vi "SUB_Calibration_by_KH_170117.vi"(11 "Test Data table":string[][](table)=[["-", "-", "5", "10", "20.025", "29.975", "39.9"], ["-", "-", "-", "-", "-", "-", "-"], ["-", "-", "-", "-", "-", "-", "-"], ["-", "-", "-", "-", "-", "-", "-"], ["-", "-", "109.9", "248.8", "515.2", "773.0", "1024.30"], ["-", "-", "-", "-", "-", "-", "-"], ["-", "-", "-", "-", "-", "-", "-"], ["-", "-", "-", "-", "-", "-", "-"], ["-", "-", "59.10", "162.20", "378.80", "615.60", "863.10"]]) -> (2 "Calibration Parameter-R":T1 {"lb offset" format="%#_13g"; "y intercept" format="%#_13g"; "Scale" format="%#_13g"; "Linear fit" format="%#_13g"}, 3 "Calibration Parameter-L":T1 {"lb offset" format="%#_13g"; "y intercept" format="%#_13g"; "Scale" format="%#_13g"; "Linear fit" format="%#_13g"})   [LabVIEW 2015]
uses:
  <vilib>/Analysis/6fits.llb/Curve Fitting Criteria.ctl
  <vilib>/Analysis/NI_AALPro.lvlib
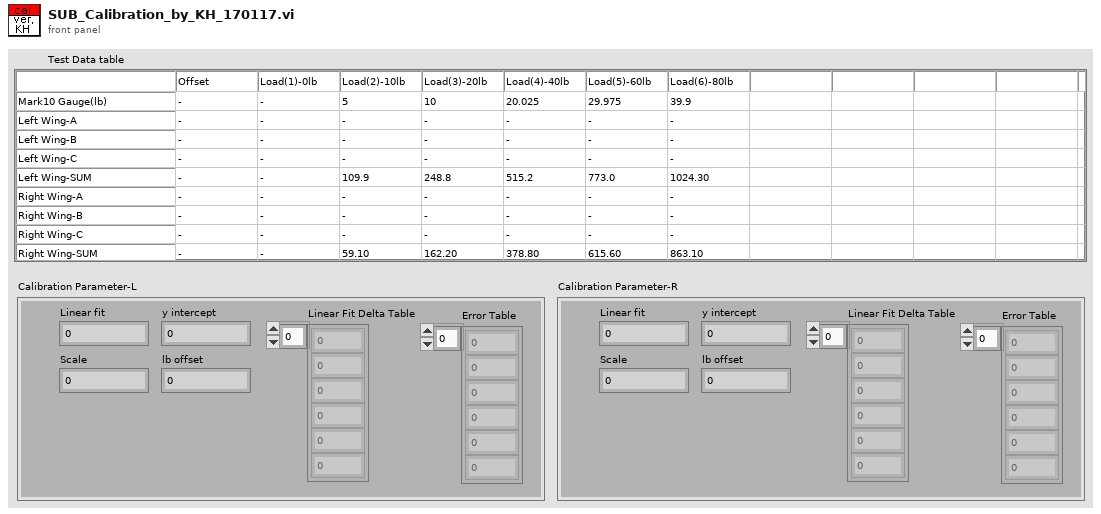
[diagram p1: front panel]
types:
  T1 = cluster{"Linear fit":dbl, "Scale":dbl, "Error Table":dbl[], "y intercept":dbl, "lb offset":dbl, "Linear Fit Delta Table":dbl[]}
  T2 = typedef "NI_AALPro.lvlib/Curve Fitting Criteria.ctl" = u16
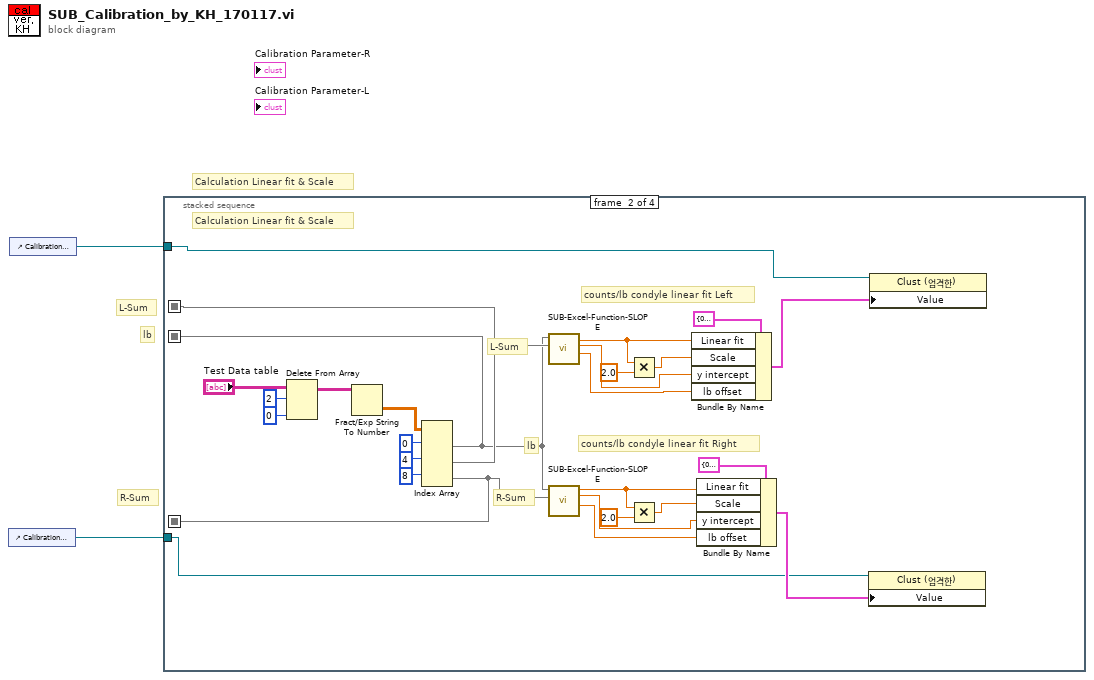
[diagram p0: block diagram]
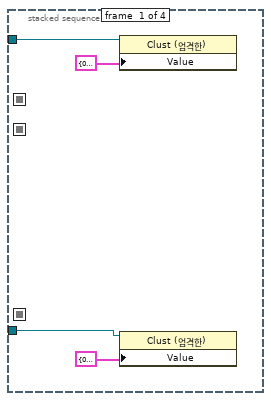
[diagram p2: hidden frame]
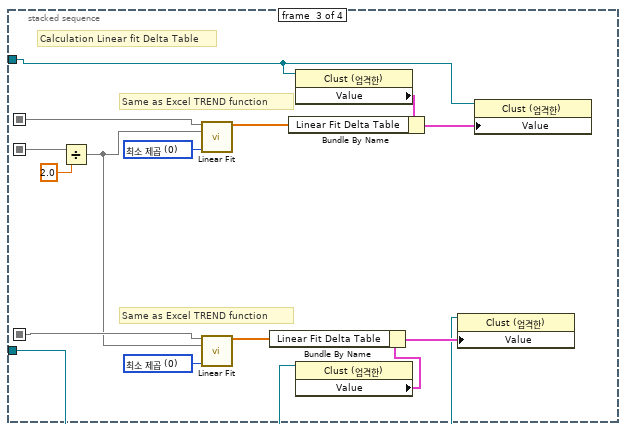
[diagram p3: hidden frame]
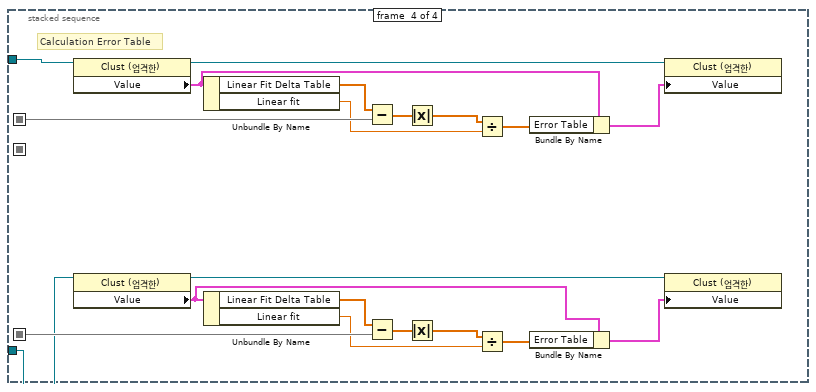
[diagram p4: hidden frame]
diagram:
  # "Calculation Linear fit & Scale"
  # "lb"
  # "R-Sum"
  # "L-Sum"
  n1 = control-ref of="Calibration Parameter-R"() -> (w1:refnum<vi>)
  n2 = control-ref of="Calibration Parameter-L"() -> (w2:refnum<vi>)
  n3 = stacked-sequence {
    seq-local: [_ w16 _ _] -> [_ _ w47 w68]
    seq-local: [_ w15 _ _] -> [_ _ w40 w67]
    seq-local: [_ w14 _ _] -> [_ _ w46 _]
    tunnel: w2 -> [w6 w13 w37 w66]
    tunnel: w1 -> [w3 w12 w35 w65]
    frame #0 {
      n4 = property class="Clust (엄격한)"(reference=w6, "Value"=T1 {"Linear fit"=0.0, "Scale"=0.0, "Error Table"=[], "y intercept"=0.0, "lb offset"=0.0, "Linear Fit Delta Table"=[]} ("Calibration Parameter-L")) -> ()  [unwired: 1 in, 2 out]
      n5 = property class="Clust (엄격한)"(reference=w3, "Value"=T1 {"Linear fit"=0.0, "Scale"=0.0, "Error Table"=[], "y intercept"=0.0, "lb offset"=0.0, "Linear Fit Delta Table"=[]} ("Calibration Parameter-L")) -> ()  [unwired: 1 in, 2 out]
    }
    frame #1 {
      # "Calculation Linear fit & Scale"
      # "counts/lb condyle linear fit Right"
      # "counts/lb condyle linear fit Left"
      # "R-Sum"
      # "L-Sum"
      # "lb"
      n6 = Delete From Array(array="Test Data table", length=2 ("길이"), index (col)=0 ("비활성화된 인덱스 (열)")) -> (array with subset deleted=w27:string[][])  [unwired: 1 in, 1 out]
      n7 = Fract/Exp String To Number(string=w27) -> (number=w26:dbl[][])  [unwired: 3 in, 1 out]
      n8 = Index Array(array=w26, index (row) #1=0 ("인덱스 (행)"), index (row) #2=4 ("인덱스 (행)"), index (row) #3=8 ("인덱스 (행)")) -> (element #1=w14:dbl[], element #2=w16:dbl[], element #3=w15:dbl[])  [unwired: 3 in]
      n9 = call "SUB-Excel-Function-SLOPE.vi"("Y"=w16, "X"=w14) -> ("offset"=w9:dbl, "intercept"=w10:dbl, "slope"=w11:dbl)  [unwired: 7 in]
      n10 = call "SUB-Excel-Function-SLOPE.vi"("Y"=w15, "X"=w14) -> ("offset"=w7:dbl, "intercept"=w8:dbl, "slope"=w17:dbl)  [unwired: 7 in]
      n11 = Multiply(x=w11, y=2.0) -> (x*y=w20:dbl)
      n12 = Multiply(x=w17, y=2.0) -> (x*y=w18:dbl)
      n13 = Bundle By Name(cluster=T1 {"Linear fit"=0.0, "Scale"=0.0, "Error Table"=[], "y intercept"=0.0, "lb offset"=0.0, "Linear Fit Delta Table"=[]} ("Calibration Parameter-L"), "Linear fit"=w11, "Scale"=w20, "y intercept"=w10, "lb offset"=w9) -> (w24:T1)
      n14 = Bundle By Name(cluster=T1 {"Linear fit"=0.0, "Scale"=0.0, "Error Table"=[], "y intercept"=0.0, "lb offset"=0.0, "Linear Fit Delta Table"=[]} ("Calibration Parameter-L"), "Linear fit"=w17, "Scale"=w18, "y intercept"=w8, "lb offset"=w7) -> (w23:T1)
      n15 = property class="Clust (엄격한)"(reference=w12, "Value"=w23) -> ()  [unwired: 1 in, 2 out]
      n16 = property class="Clust (엄격한)"(reference=w13, "Value"=w24) -> ()  [unwired: 1 in, 2 out]
    }
    frame #2 {
      w41 = T2 0 items=["최소 제곱", "최소 절대 오차", "바이스퀘어(Bisquare)"] ("method")
      w48 = T2 0 items=["최소 제곱", "최소 절대 오차", "바이스퀘어(Bisquare)"] ("method")
      # "Calculation Linear fit Delta Table"
      # "Same as Excel TREND function"
      # "Same as Excel TREND function"
      n17 = Divide(x=w46, y=2.0) -> (x/y=w39:dbl[])
      n18 = call <vilib>:"Linear Fit.vi"("Y"=w47, "X"=w39, "method"=w48) -> ("Best Linear Fit"=w44:dbl[])  [unwired: 8 in, 4 out]
      n19 = call <vilib>:"Linear Fit.vi"("Y"=w40, "X"=w39, "method"=w41) -> ("Best Linear Fit"=w42:dbl[])  [unwired: 8 in, 4 out]
      n20 = property class="Clust (엄격한)"(reference=w37) -> ("Value"=w36:T1)  [unwired: 1 in, 2 out]
      n21 = Bundle By Name(cluster=w36, "Linear Fit Delta Table"=w44) -> (w38:T1)
      n22 = property class="Clust (엄격한)"(reference=w35) -> ("Value"=w34:T1)  [unwired: 1 in, 2 out]
      n23 = Bundle By Name(cluster=w34, "Linear Fit Delta Table"=w42) -> (w43:T1)
      n24 = property class="Clust (엄격한)"(reference=w35, "Value"=w43) -> ()  [unwired: 1 in, 2 out]
      n25 = property class="Clust (엄격한)"(reference=w37, "Value"=w38) -> ()  [unwired: 1 in, 2 out]
    }
    frame #3 {
      # "Calculation Error Table"
      n26 = property class="Clust (엄격한)"(reference=w66) -> (reference out=w51:refnum<vi>, "Value"=w50:T1)  [unwired: 1 in, 1 out]
      n27 = property class="Clust (엄격한)"(reference=w65) -> (reference out=w56:refnum<vi>, "Value"=w49:T1)  [unwired: 1 in, 1 out]
      n28 = Unbundle By Name(w50) -> ("Linear Fit Delta Table"=w64:dbl[], "Linear fit"=w61:dbl)
      n29 = Unbundle By Name(w49) -> ("Linear Fit Delta Table"=w52:dbl[], "Linear fit"=w55:dbl)
      n30 = Subtract(x=w64, y=w68) -> (x-y=w63:dbl[])
      n31 = Subtract(x=w52, y=w67) -> (x-y=w53:dbl[])
      n32 = Absolute Value(x=w63) -> (abs(x)=w62:dbl[])
      n33 = Absolute Value(x=w53) -> (abs(x)=w54:dbl[])
      n34 = Divide(x=w62, y=w61) -> (x/y=w60:dbl[])
      n35 = Divide(x=w54, y=w55) -> (x/y=w57:dbl[])
      n36 = Bundle By Name(cluster=w50, "Error Table"=w60) -> (w59:T1)
      n37 = Bundle By Name(cluster=w49, "Error Table"=w57) -> (w58:T1)
      n38 = property class="Clust (엄격한)"(reference=w51, "Value"=w59) -> ()  [unwired: 1 in, 2 out]
      n39 = property class="Clust (엄격한)"(reference=w56, "Value"=w58) -> ()  [unwired: 1 in, 2 out]
    }
  }
